vi "graph Size change (SubVI).vi"(10 "Plot Area Size in":T1, 11 "Boolean in":refnum<vi>) -> (2 "Plot Area Size out":T1, 4 "Value":bool)   [LabVIEW 2013]
uses:
  <vilib>/Utility/miscctls.llb/LVBoundsTypeDef.ctl
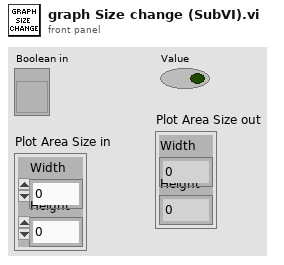
[diagram p1: front panel]
types:
  T1 = typedef "LVBoundsTypeDef.ctl" = cluster{"Width":u32, "Height":u32}
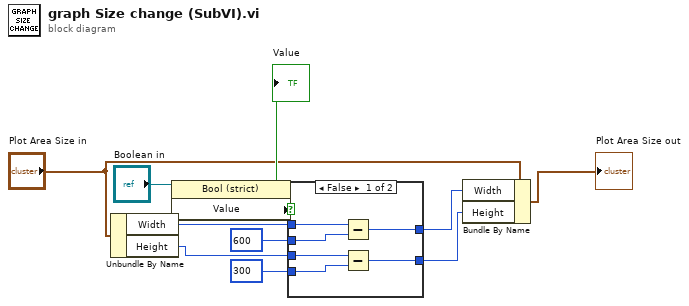
[diagram p0: block diagram]
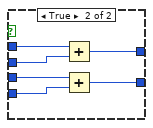
[diagram p2: hidden frame]
diagram:
  n1 = Unbundle By Name("Plot Area Size in") -> ("Width"=w5:u32, "Height"=w3:u32)
  n2 = property on="Property Node" class="Bool (strict)"(reference="Boolean in") -> ("Value"=w10:bool)  [unwired: 1 in, 2 out]
  "Value" <- w10
  n3 = case shown="False" w10 {
    tunnel: w5 -> [w16 w22]
    tunnel: [w15 w21] -> w4
    tunnel: w3 -> [w14 w20]
    tunnel: [w13 w19] -> w2
    tunnel: u32 300 ("y") -> [w11 w18]
    tunnel: u32 600 ("y 2") -> [w12 w17]
    frame False {
      n4 = Subtract(x=w16, y=w12) -> (x-y=w15:u32)
      n5 = Subtract(x=w14, y=w11) -> (x-y=w13:u32)
    }
    frame True {
      n6 = Add(x=w22, y=w17) -> (x+y=w21:u32)
      n7 = Add(x=w20, y=w18) -> (x+y=w19:u32)
    }
  }
  n8 = Bundle By Name(cluster="Plot Area Size in", "Width"=w4, "Height"=w2) -> (→"Plot Area Size out":T1)
